vi "Get Picture.vi"(8 "error in (no error)":errorcluster, 11 "Metal in":refnum<class "Metal.lvclass">) -> (0 "error out":errorcluster, 2 "Picture":picture, 3 "Metal out":refnum<class "Metal.lvclass">)   [LabVIEW 2020, in "Metal.lvclass"]
uses:
  Metal.lvclass
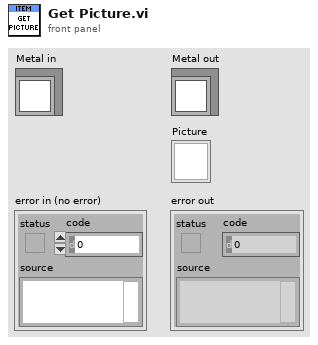
[diagram p1: front panel]
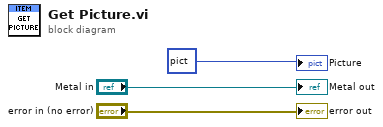
[diagram p0: block diagram]
diagram:
  "error out" <- "error in (no error)"
  "Metal out" <- "Metal in"
  "Picture" <- picture bytes[3230] ("new picture")
